vi "Tester 1.vi"() -> ()   [LabVIEW 2023, in "Error Manager.lvlib" / "Error Display Window.lvclass"]
doc: "Tester 1"
uses:
  Error Display Window.lvclass
  Error Details (cluster).ctl
  6d855587-16f8-4686-8f82-444d98388444.vi
  b33024f9-6de8-41ee-ba7d-9a2c31ef14c5.vi
panel:
  out "Error Out":errorcluster
  # "Tester 1"
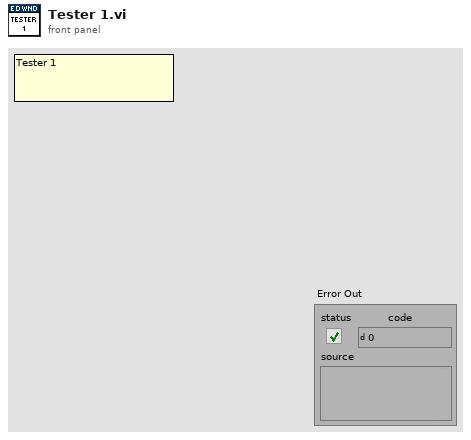
[diagram p1: front panel]
types:
  T1 = typedef "Error Manager.lvlib/Error Display Window.lvclass/Error Details (cluster).ctl" = cluster{"Error Code":i32, "Error Message":string, "Error Timestamp":timestamp}
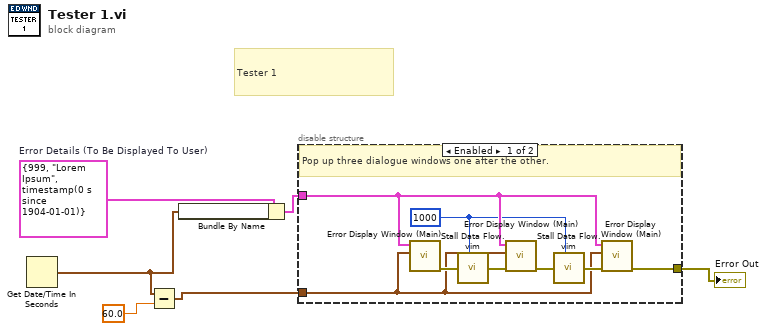
[diagram p0: block diagram]
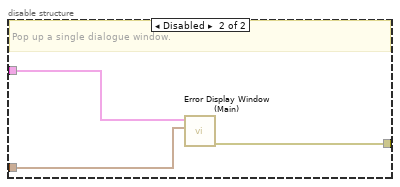
[diagram p2: hidden frame]
diagram:
  w5 = T1 {"Error Code"=999, "Error Message"="Lorem Ipsum", "Error Timestamp"=timestamp(0 s since 1904-01-01)}  # Error Details (To Be Displayed To User)
  # "Tester 1"
  n1 = Get Date/Time In Seconds() -> (seconds since 1Jan1904=w3:timestamp)
  n2 = Subtract(x=w3, y=60.0) -> (x-y=w1:timestamp)
  n3 = Bundle By Name(cluster=w5, w3) -> (w4:T1)
  n4 = disable-structure shown="Enabled" {
    disable-tunnel: [w10 w17] -> w6
    disable-tunnel: w4 -> [w9 w16]
    disable-tunnel: w1 -> [w7 w15]
    frame Enabled {
      w8 = u32 1000 ("milliseconds to wait")
      # "Pop up three dialogue windows one after the other."
      n5 = call "Error Display Window (Main).vi"(10:w7, 11:w9) -> (0:w14:errorcluster)  [unwired: 9 in]
      n6 = call "Stall Data Flow.vim"(0:w14, 1:w8) -> (3:w12:errorcluster)  [unwired: 1 out]
      n7 = call "Error Display Window (Main).vi"(8:w12, 10:w7, 11:w9) -> (0:w13:errorcluster)  [unwired: 8 in]
      n8 = call "Stall Data Flow.vim"(0:w13, 1:w8) -> (3:w11:errorcluster)  [unwired: 1 out]
      n9 = call "Error Display Window (Main).vi"(8:w11, 10:w7, 11:w9) -> (0:w10:errorcluster)  [unwired: 8 in]
    }
    frame Disabled {
      # "Pop up a single dialogue window."
      n10 = call "Error Display Window (Main).vi"(10:w15, 11:w16) -> (0:w17:errorcluster)  [unwired: 9 in]
    }
  }
  "Error Out" <- w6
